vi "get_and_insert_SN.vi"(8 "error in (no error)":errorcluster, 10 "read buffer in":string, 11 "VISA Refnum in":refnum<visa-resource-name>) -> (0 "error out":errorcluster, 2 "read buffer out":string, 3 "VISA Refnum out":refnum<visa-resource-name>)   [LabVIEW 2015]
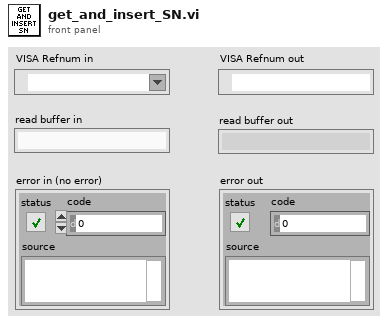
[diagram p1: front panel]
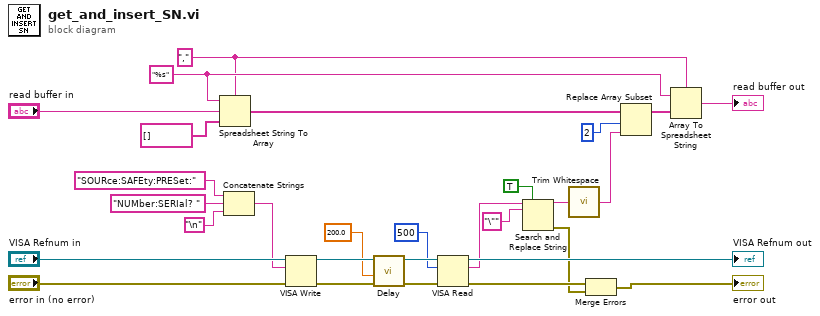
[diagram p0: block diagram]
diagram:
  w26 = "," ("delimiter (Tab)")
  w27 = "%s" ("format string")
  n1 = Spreadsheet String To Array(delimiter (Tab)=w26, format string=w27, spreadsheet string="read buffer in", array type (2D Dbl)=string[] []) -> (array=w16:string[])
  n2 = Concatenate Strings("SOURce:SAFEty:PRESet:", "NUMber:SERIal? ", "\n") -> (w7:string)
  n3 = VISA Write(VISA resource name="VISA Refnum in", write buffer=w7, error in (no error)="error in (no error)") -> (VISA resource name out=w28:refnum<visa-resource-name>, error out=w4:errorcluster)  [unwired: 1 out]
  n4 = call "Delay.vi"("error in (no error)"=w4, "milliseconds to wait"=200.0) -> ("error out"=w5:errorcluster)  [unwired: 9 in]
  n5 = VISA Read(VISA resource name=w28, byte count=u32 500, error in (no error)=w5) -> (VISA resource name out=→"VISA Refnum out":refnum<visa-resource-name>, read buffer=w8:string, error out=w21:errorcluster)  [unwired: 1 out]
  n6 = Search and Replace String(replace all?=TRUE ("replace all? (F)"), input string=w8, search string="\"" ("substring (\"\")")) -> (result string=w18:string, error out=w1:errorcluster)  [unwired: 5 in, 2 out]
  n7 = call <vilib>:"Trim Whitespace.vi"("string"=w18) -> ("trimmed string"=w25:string)  [unwired: 1 in]
  n8 = Merge Errors(w21, w1) -> (→"error out":errorcluster)
  n9 = Replace Array Subset(array=w16, new element=w25, index=2) -> (w23:string[])
  n10 = Array To Spreadsheet String(delimiter (Tab)=w26, array=w23, 3:w27) -> (spreadsheet string=→"read buffer out":string)
